vi "BundleMagic TEST.vi"() -> ()   [LabVIEW 2023]
uses:
  <vilib>/Utility/miscctls.llb/LVBoundsTypeDef.ctl
panel:
  out "Cluster with unnamed elements 2":T1
  in  "Single Element Cluster":cluster{"Numeric":dbl}
  in  "Cluster with unnamed elements":T2
  in  "Cluster with Dotted Names":T3 {"C1.1"."N2.2" format="%.3p"}
  out "Bounds":T4
  out "Owner":refnum<vi>
  in  "Cluster":T5 {"C1"."N2" format="%.3p"}
  # "Dummy controls for use on BD"
  # "BundleMag!c FP Actions"
  # "Select Classes via Browse Classes... dialog on this control"
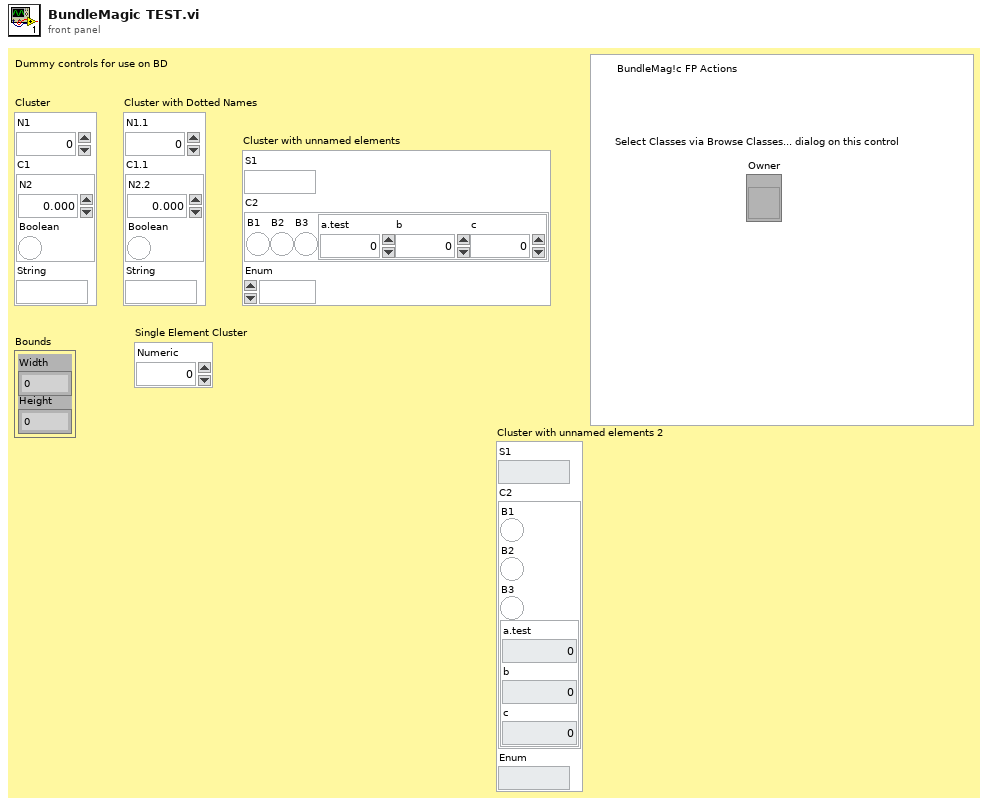
[diagram p1: front panel]
types:
  T1 = cluster{"S1":string, "C2":cluster{"B1":bool, "B2":bool, "B3":bool, "Cluster":cluster{"a.test":dbl, "b":i32, "c":u8}}, "Enum":enum16{""}}
  T2 = cluster{"S1":string, "C2":cluster{"B1":bool, "B2":bool, "B3":bool, cluster{"a.test":dbl, "b":i32, "c":u8}}, "Enum":enum16{""}}
  T3 = cluster{"N1.1":dbl, "C1.1":cluster{"N2.2":dbl, "Boolean":bool}, "String":string}
  T4 = typedef "LVBoundsTypeDef.ctl" = cluster{"Width":u32, "Height":u32}
  T5 = cluster{"N1":dbl, "C1":cluster{"N2":dbl, "Boolean":bool}, "String":string}
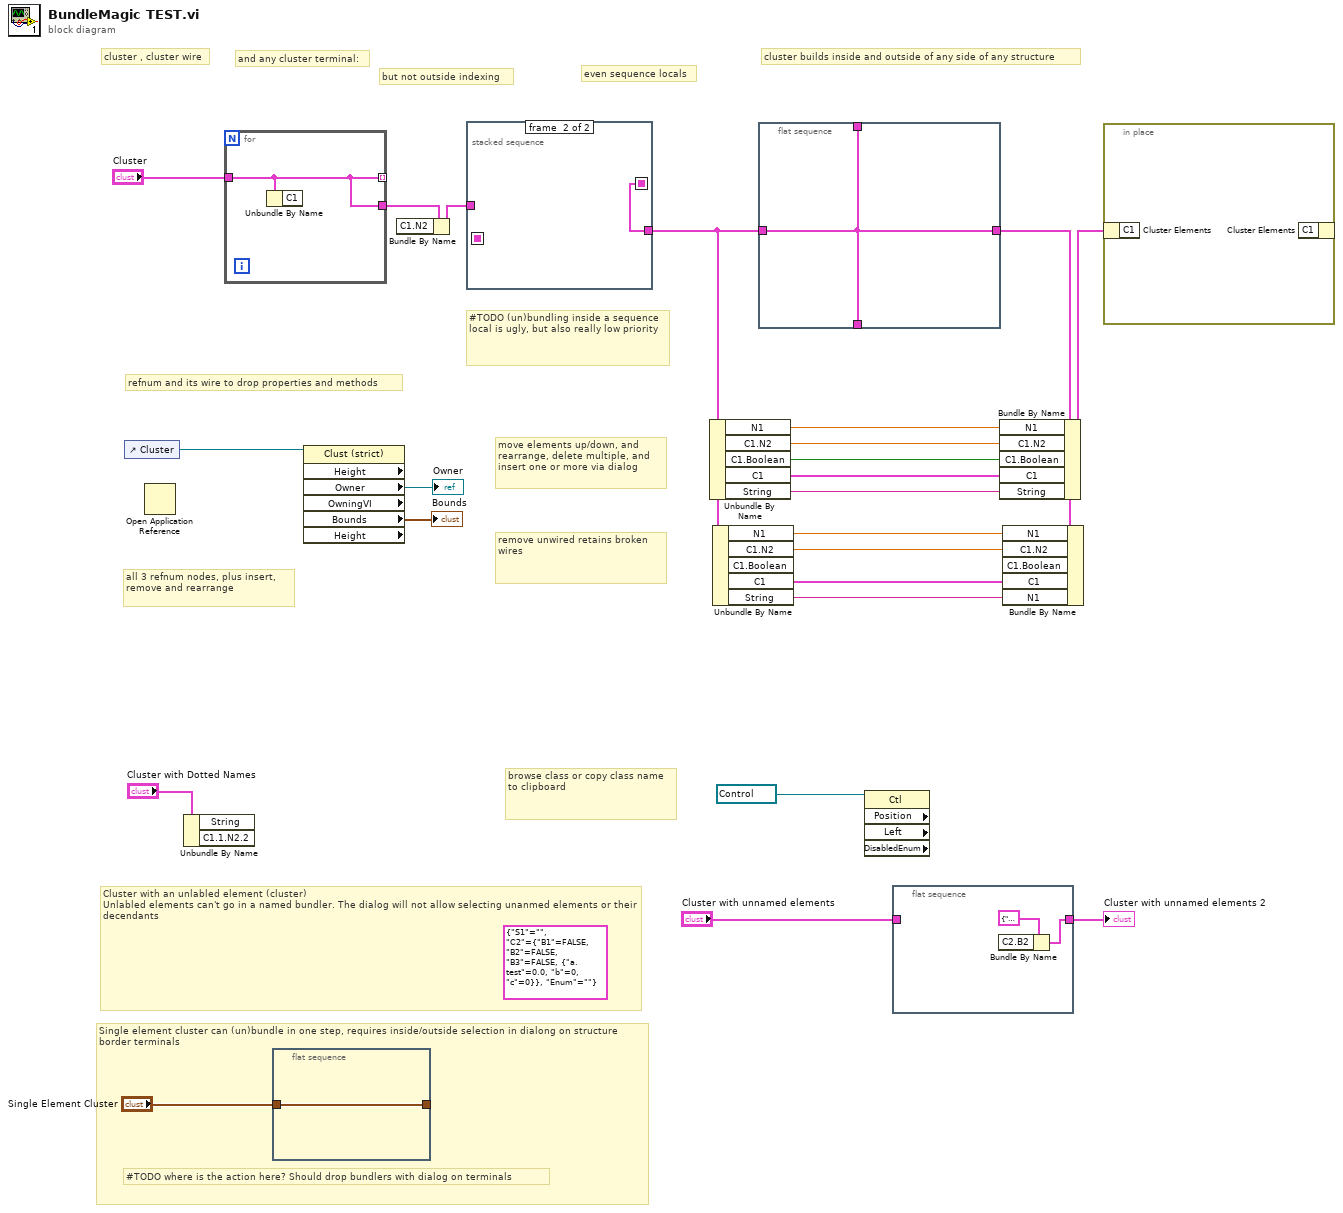
[diagram p0: block diagram]
diagram:
  (unwired) T2 {"S1"="", "C2"={"B1"=FALSE, "B2"=FALSE, "B3"=FALSE, {"a.test"=0.0, "b"=0, "c"=0}}, "Enum"=enum.""} ("C1")
  # "#TODO where is the action here? Should drop bundlers with dialog on terminals"
  # "browse class or copy class name to clipboard"
  # "remove unwired retains broken wires"
  # "move elements up/down, and rearrange, delete multiple, and insert one or more via dialog"
  # "#TODO (un)bundling inside a sequence local is ugly, but also really low priority"
  # "even sequence locals"
  # "but not outside indexing"
  # "and any cluster terminal:"
  # "cluster , cluster wire"
  # "cluster builds inside and outside of any side of any structure"
  # "refnum and its wire to drop properties and methods"
  # "all 3 refnum nodes, plus insert, remove and rearrange"
  # "Cluster with an unlabled element (cluster)\nUnlabled elements can't go in a named bundler. The dialog will not allow selecting unanmed elements or their decendants"
  # "Single element cluster can (un)bundle in one step, requires inside/outside selection in dialong on structure border terminals"
  n1 = control-ref of="Cluster"() -> (w9:refnum<vi>)
  n2 = Open Application Reference() -> ()  [unwired: 4 in, 2 out]
  n3 = Unbundle By Name("Cluster with Dotted Names") -> ()  [unwired: 2 out]
  n4 = for {
    tunnel: [w25] -> _ mode=indexing
    tunnel: "Cluster" -> [w25]
    tunnel: [w25] -> w24
    n5 = Unbundle By Name(w25) -> ()  [unwired: 1 out]
  }
  n6 = flat-sequence {
    tunnel: [w26] -> _
    tunnel: "Single Element Cluster" -> [w26]
    frame #0 {
    }
  }
  n7 = property class="Clust (strict)" props=["Height", "Owner", "OwningVI", "Bounds", "Height"](reference=w9) -> ("Owner"=→"Owner":refnum<vi>, "Bounds"=→"Bounds":T4, "Height"=w8:u32)  [unwired: 1 in, 4 out]
  n8 = Bundle By Name(cluster=w24) -> (w12:T5)  [unwired: 1 in]
  n9 = stacked-sequence {
    seq-local: [w27 _] -> [_ w28]
    seq-local: [w27 _] -> [_ _]
    tunnel: w12 -> [w27 _]
    tunnel: [_ w28] -> w4
    frame #0 {
    }
    frame #1 {
    }
  }
  n10 = Unbundle By Name(w4) -> ("N1"=w22:dbl, "C1.N2"=w21:dbl, "C1.Boolean"=w19:bool, "C1"=w20:cluster{"N2":dbl, "Boolean":bool}, "String"=w18:string)
  n11 = Unbundle By Name(w4) -> ("N1"=w15:dbl, "C1.N2"=w16:dbl, "C1"=w17:cluster{"N2":dbl, "Boolean":bool}, "String"=w5:string)  [unwired: 1 out]
  n12 = flat-sequence {
    tunnel: [w29] -> _
    tunnel: w4 -> [w29]
    tunnel: [w29] -> _
    tunnel: [w29] -> w3
    frame #0 {
    }
  }
  n13 = property class="Ctl" props=["Position", "Left", "DisabledEnum"](reference=refnum<vi> refnum ("Owner")) -> ()  [unwired: 1 in, 5 out]
  n14 = flat-sequence {
    tunnel: [w31] -> w6
    tunnel: "Cluster with unnamed elements" -> [_]
    frame #0 {
      n15 = Bundle By Name(cluster=T2 {"S1"="", "C2"={"B1"=FALSE, "B2"=FALSE, "B3"=FALSE, {"a.test"=0.0, "b"=0, "c"=0}}, "Enum"=enum.""} ("Cluster with unnamed elements")) -> (w31:T2)  [unwired: 1 in]
    }
  }
  n16 = Bundle By Name(cluster=w3, "N1"=w22, "C1.N2"=w21, "C1.Boolean"=w19, "C1"=w20, "String"=w18) -> (w23:T5)
  n17 = Bundle By Name(cluster=w3, "N1"=w15, "C1.N2"=w16, "C1"=w17, "N1"=w5) -> ()  [unwired: 1 in, 1 out]
  n18 = in-place {
    n19 = in-place-cluster #1(w23) -> ()  [unwired: 1 out]
    n20 = in-place-cluster #1() -> ()  [unwired: 1 in, 1 out]
  }
  "Cluster with unnamed elements 2" <- w6
